vi "GenerateDataSet.vi"(11 "Records":i32) -> (3 "DataGrid":string[][](array[string]))   [LabVIEW 2016, in "DataGrid.lvlib" / "DataGridView.lvclass"]
uses:
  <userlib>/LabVIEWdotNetDataGrid/source/DataGridView/DataGridView.lvclass
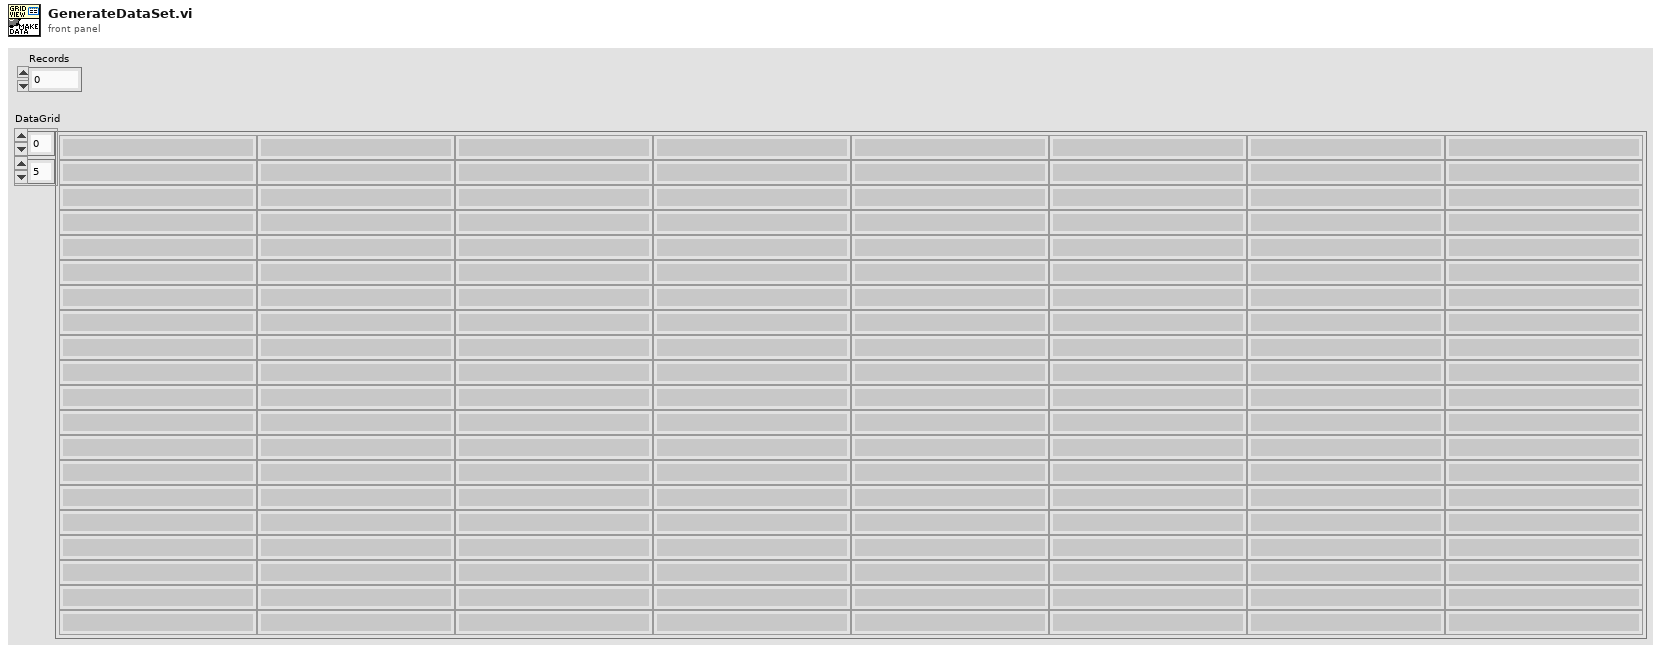
[diagram p1: front panel]
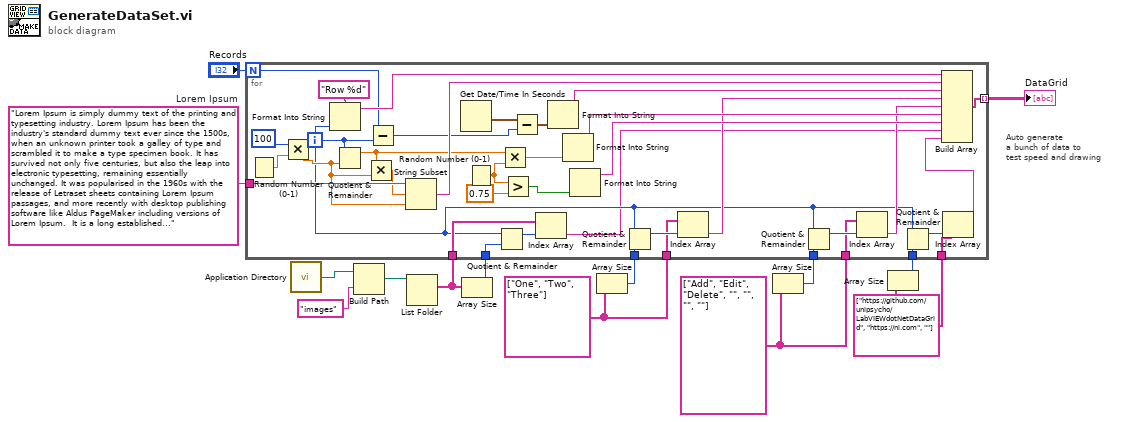
[diagram p0: block diagram]
diagram:
  w2 = string[] ["https://github.com/unipsycho/LabVIEWdotNetDataGrid", "https://ni.com", ""]
  w4 = string[] ["Add", "Edit", "Delete", "", "", "", ""]
  w6 = string[] ["One", "Two", "Three"]
  w9 = "Lorem Ipsum is simply dummy text of the printing and typesetting industry. Lorem Ipsum has been the industry's standard dummy text ever since the 1500s, when an unknown printer took a galley of type and scrambled it to make a type specimen book. It has survived not only five centuries, but also the leap into electronic typesetting, remaining essentially unchanged. It was popularised in the 1960s with the release of Letraset sheets containing Lorem Ipsum passages, and more recently with desktop publishing software like Aldus PageMaker including versions of Lorem Ipsum.  It is a long established fact that a reader will be distracted by the readable content of a page when looking at its layout. The point of using Lorem Ipsum is that it has a more-or-less normal distribution of letters, as opposed to using 'Content here, content here', making it look like readable English. Many desktop publishing packages and web page editors now use Lorem Ipsum as their default model text, and a search for 'lorem ipsum' will uncover many web sites still in their infancy. Various versions have evolved over the years, sometimes by accident, sometimes on purpose (injected humour and the like). Contrary to popular belief, Lorem Ipsum is not simply random text. It has roots in a piece of classical Latin literature from 45 BC, making it over 2000 years old. Richard McClintock, a Latin professor at Hampden-Sydney College in Virginia, looked up one of the more obscure Latin words, consectetur, from a Lorem Ipsum passage, and going through the cites of the word in classical literature, discovered the undoubtable source. Lorem Ipsum comes from sections 1.10.32 and 1.10.33 of \"de Finibus Bonorum et Malorum\" (The Extremes of Good and Evil) by Cicero, written in 45 BC. This book is a treatise on the theory of ethics, very popular during the Renaissance. The first line of Lorem Ipsum, \"Lorem ipsum dolor sit amet..\", comes from a line in section 1.10.32. The standard chunk of Lorem Ipsum used since the 1500s is reproduced below for those interested. Sections 1.10.32 and 1.10.33 from \"de Finibus Bonorum et Malorum\" by Cicero are also reproduced in their exact original form, accompanied by English versions from the 1914 translation by H. Rackham. There are many variations of passages of Lorem Ipsum available, but the majority have suffered alteration in some form, by injected humour, or randomised words which don't look even slightly believable. If you are going to use a passage of Lorem Ipsum, you need to be sure there isn't anything embarrassing hidden in the middle of text. All the Lorem Ipsum generators on the Internet tend to repeat predefined chunks as necessary, making this the first true generator on the Internet. It uses a dictionary of over 200 Latin words, combined with a handful of model sentence structures, to generate Lorem Ipsum which looks reasonable. The generated Lorem Ipsum is therefore always free from repetition, injected humour, or non-characteristic words etc."  # Lorem Ipsum
  # "Auto generate\na bunch of data to \ntest speed and drawing"
  n1 = call <vilib>:"Application Directory.vi"() -> ("Application Directory"=w1:path)
  n2 = Build Path(base path=w1, name or relative path="images") -> (appended path=w12:path)
  n3 = List Folder(path=w12) -> (filenames=w13:string[])  [unwired: 3 in, 3 out]
  n4 = Array Size(array=w13) -> (size(s)=w14:i32)
  n5 = Array Size(array=w6) -> (size(s)=w7:i32)
  n6 = Array Size(array=w4) -> (size(s)=w5:i32)
  n7 = Array Size(array=w2) -> (size(s)=w3:i32)
  n8 = for {
    N: "Records" -> [w45]
    tunnel: [w50] -> w8 mode=indexing
    tunnel: w9 -> [w49]
    tunnel: w13 -> [w34]
    tunnel: w14 -> [w16]
    tunnel: w6 -> [w31]
    tunnel: w7 -> [w30]
    tunnel: w5 -> [w27]
    tunnel: w4 -> [w26]
    tunnel: w3 -> [w21]
    tunnel: w2 -> [w20]
    i -> [w17]
    n9 = Random Number (0-1)() -> (number: 0 to 1=w24:dbl)
    n10 = Multiply(x=100 ("y"), y=w24) -> (x*y=w22:dbl)
    n11 = Format Into String(format string="Row %d", w17) -> (resulting string=w51:string)  [unwired: 2 in, 1 out]
    n12 = Quotient & Remainder(x=w17, y=w22) -> (x-y*floor(x/y)=w41:dbl)  [unwired: 1 out]
    n13 = Multiply(x=w41, y=w22) -> (x*y=w48:dbl)
    n14 = Subtract(x=w45, y=w17) -> (x-y=w44:i32)
    n15 = String Subset(string=w49, offset (0)=w48, length (rest)=w22) -> (substring=w47:string)
    n16 = Get Date/Time In Seconds() -> (seconds since 1Jan1904=w46:timestamp)
    n17 = Random Number (0-1)() -> (number: 0 to 1=w38:dbl)
    n18 = Quotient & Remainder(x=w17, y=w16) -> (x-y*floor(x/y)=w33:i32)  [unwired: 1 out]
    n19 = Multiply(x=w41, y=w38) -> (x*y=w40:dbl)
    n20 = Greater?(x=w38, y=0.75) -> (0:w36:bool)
    n21 = Subtract(x=w46, y=w44) -> (x-y=w43:timestamp)
    n22 = Index Array(array=w34, index=w33) -> (element=w15:string)
    n23 = Format Into String(w43) -> (resulting string=w42:string)  [unwired: 3 in, 1 out]
    n24 = Format Into String(w40) -> (resulting string=w39:string)  [unwired: 3 in, 1 out]
    n25 = Format Into String(w36) -> (resulting string=w35:string)  [unwired: 3 in, 1 out]
    n26 = Quotient & Remainder(x=w17, y=w30) -> (x-y*floor(x/y)=w32:i32)  [unwired: 1 out]
    n27 = Index Array(array=w31, index=w32) -> (element=w29:string)
    n28 = Quotient & Remainder(x=w17, y=w27) -> (x-y*floor(x/y)=w28:i32)  [unwired: 1 out]
    n29 = Index Array(array=w26, index=w28) -> (element=w25:string)
    n30 = Quotient & Remainder(x=w17, y=w21) -> (x-y*floor(x/y)=w19:i32)  [unwired: 1 out]
    n31 = Index Array(array=w20, index=w19) -> (element=w18:string)
    n32 = Build Array(w51, w47, w42, w29, w25, w39, w35, w15, w18) -> (w50:string[])
  }
  "DataGrid" <- w8
